vi "WildBugChilGru_V2.0.1.vi"() -> ()   [LabVIEW 2014]
uses:
  <vilib>/Utility/miscctls.llb/LVPointTypeDef.ctl
  <vilib>/Utility/xml.llb/Read From XML File(string).vi
  <vilib>/Utility/xml.llb/Write to XML File(string).vi
  <vilib>/Instr/_visa.llb/VISA Configure Serial Port (Instr).vi
  <vilib>/Analysis/3filter.llb/IIR Filter (DBL).vi
  <vilib>/gmath/NI_Gmath.lvlib
  <vilib>/Analysis/NI_AALBase.lvlib
panel:
  out "Hinterrad (Tacho)\n[km/h]":dbl(knob) scale=0.0..150.0 scale format="%#.0f"
  out "Welle (Tacho)\n[1/min]":cluster{dbl, dbl}(knob) scale=0.0..14000.0
  out "XY-Graph":cluster{dbl[], dbl[]}[](graph)
  in  "Registerkarte":T1(tab)
  in  "Zündung [Imp/U]":dbl=1.0
  in  "Übersetzung ermitteln aus":T2(ring)
  in  "Getriebe [1:]":dbl=4.0
  in  "Reifenumfang [m]":dbl=1.2
  in  "Dauer [s]":dbl=5.0
  in  "nKuWe/nRolle":dbl=1.0 format="%#.3f"
  in  "Lufttemperatur [°C]":dbl
  in  "Luftfeuchtigkeit [%]":dbl=43.8
  in  "Luftdruck [mbar]":dbl=1013.45
  in  "Messung Klimadaten":bool=TRUE
  in  "Gleitender Mittelwert":u8=35
  in  "Differenzenquotient":u8=12
  in  "n vom Gas [1/min]":dbl=5000.0
  in  "Rollengeber [Inkr/U]":u16=200
  in  "Rollenumfang [m]":dbl=0.613
  in  "Rollenträgheit [kgm²]":dbl=0.402
  in  "Recalc":bool
  in  "Leistung":bool=TRUE caption="Messung Klimadaten"
  in  "Ende":bool
  out "Datenspeicher":T3={"Fahrzeugdaten"="", "date/time string"="", "Rolle [Inkr/U]"=200, "Rollenumfang [m]"=0.613, "Rollenträgheit [kgm²]"=0.402, "Zündung [Imp/U]"=1.0, "Getriebe [1:]"=4.0, "Reifenumfang [m] "=1.2, "element"=0.0, "Gl. Mittelwert"=35, "Differenzenquotient"=12, "Polynom"=0, "dT [s]"=0.0, "element"=0.0, "Lufttemperatur [°C]"=0.0, "Luftfeuchtigkeit [%]"=43.8, "Luftdruck [mbar]"=1013.45, [], [], "Best Polynomial Fit"=[], [], "Übersetzung ermitteln aus"=0, "[s]"=5.0, "nmin [1/min]"=0.0, "nmax [1/min]"=0.0, "n vom Gas [1/min]"=5000.0, "dT-Array [s]"=[], [], "Boolesch"=TRUE, "Serielle Schnittstelle"="COM6", "nKuWe/nRolle"=1.0}
  out "COM-Fehlerrate":string="0 / 0,0%"
  in  "Konfiguration:":bool
  in  "Speichern":bool
  in  "Drucken":bool
  out "Pmax":string="0,0 PS"
  out "Ergebnis":string
  in  "Fahrzeugdaten":string
  out "Untersetzung\nermittelt":bool
  out "Untersetzung":dbl format="%#.3f"
  in  "Start":bool
  out "Füllstand Lesepuffer":u64(slide)=1 scale=1.0..100.0
  out "Hinterrad\n[km/h]":dbl(knob) scale=0.0..150.0
  out "Welle\n[1/min]":cluster{dbl, dbl}(knob) scale=0.0..14000.0
  out "Lesepuffer":string="\n"
  in  "Serielle Schnittstelle":refnum<visa-resource-name>="COM6"
  out "Untersetzung-Graph":dbl(graph)=198.99999999999997 caption="Untersetzung"
  # "1. n konstant halten\n2. START\n3. n weiter halten\n4. bei GO: Vollgas\n5. vom Gas gehen"
  # "Zündung\nRolle"
  # "Zündung\nRolle"
  # "Untersetzung aus:"
  # "Eingabe <> Messen"
  # "Tacho <> Leistung"
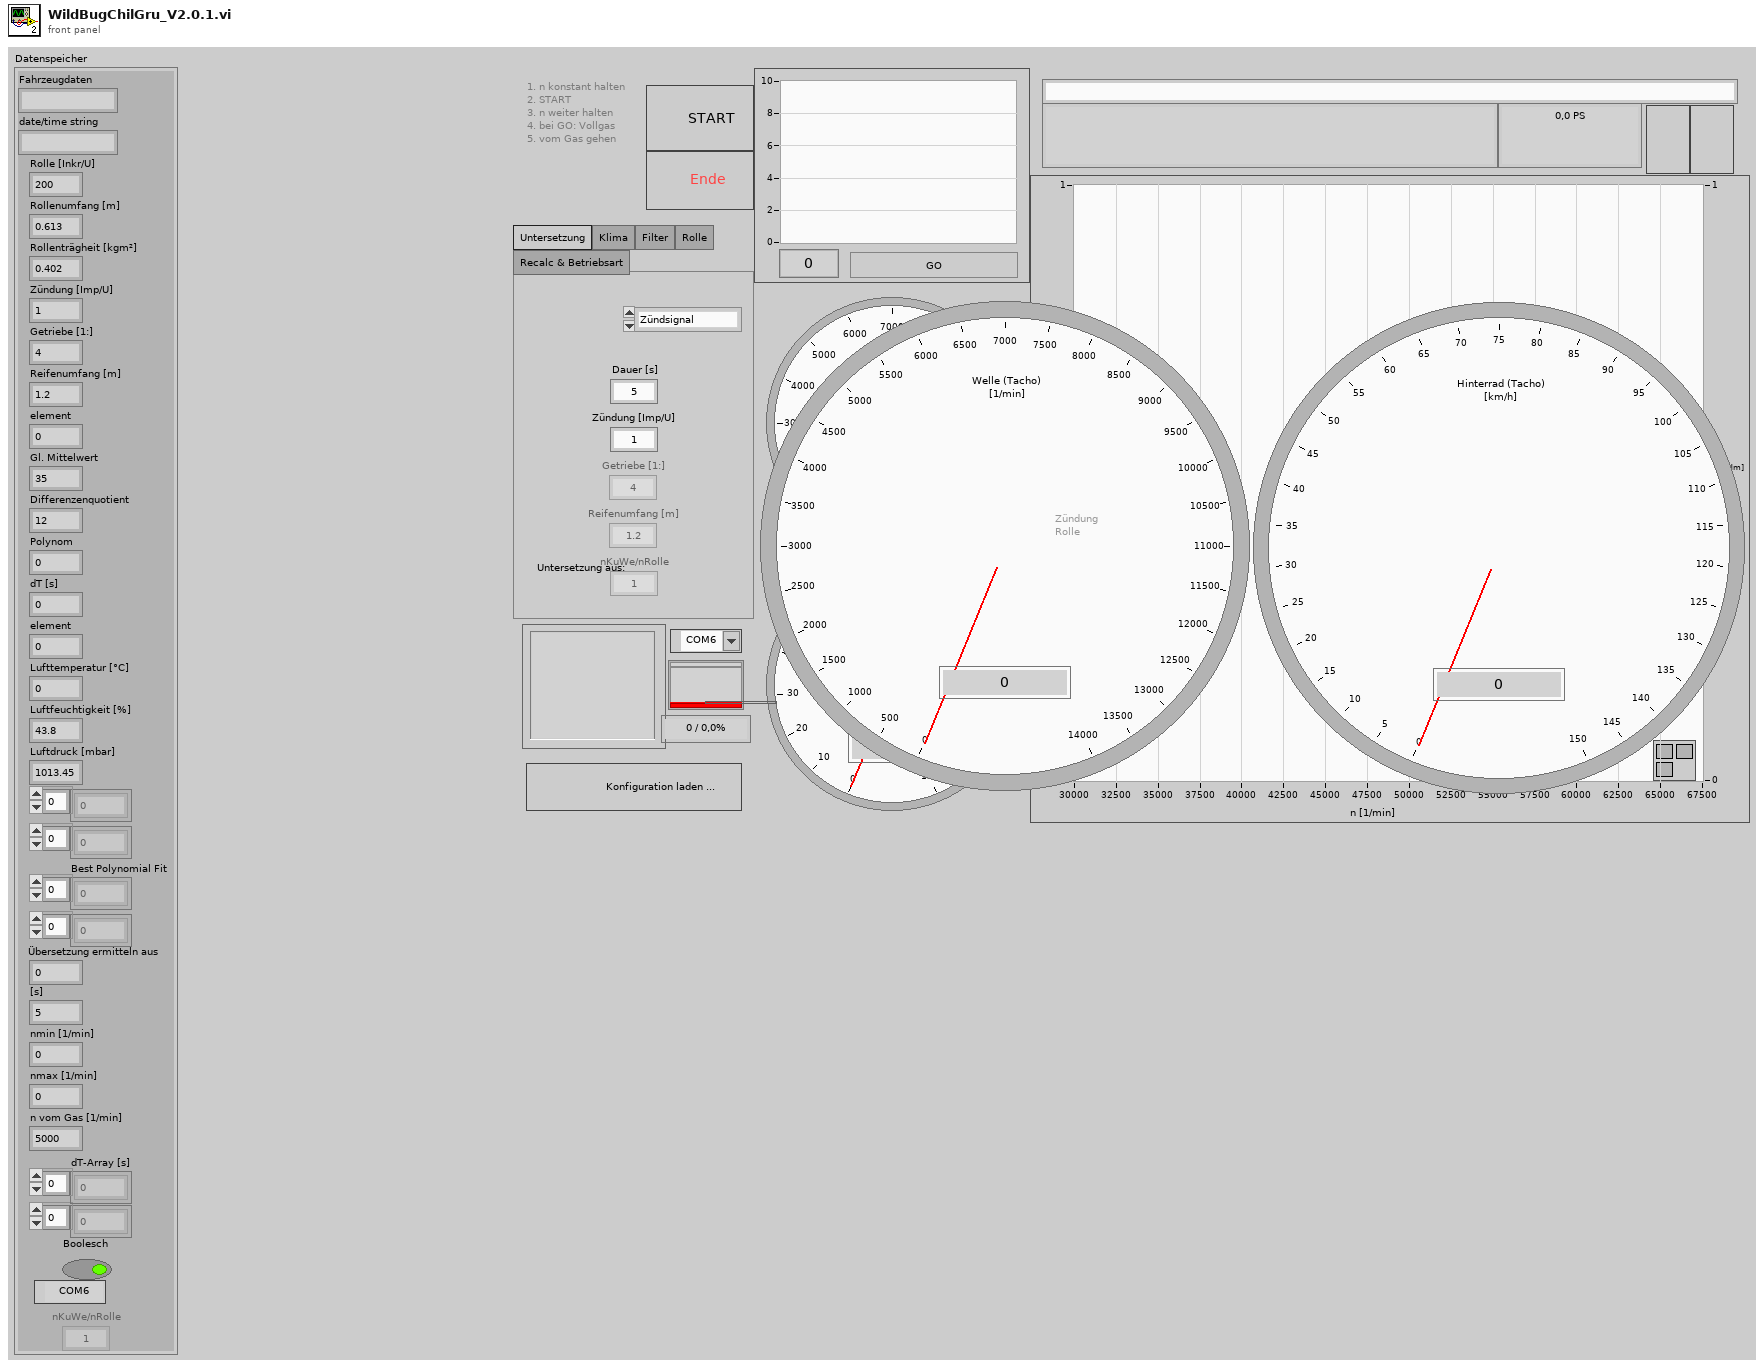
[diagram p1: front panel]
types:
  T1 = enum32{"Untersetzung", "Klima", "Filter", "Rolle", "Recalc & Betriebsart"}
  T2 = enum8{"Zündsignal", "Getriebe & Reifen", "nKuWe / nRolle"}
  T3 = cluster{"Fahrzeugdaten":string, "date/time string":string, "Rolle [Inkr/U]":u16, "Rollenumfang [m]":dbl, "Rollenträgheit [kgm²]":dbl, "Zündung [Imp/U]":dbl, "Getriebe [1:]":dbl, "Reifenumfang [m] ":dbl, "element":dbl, "Gl. Mittelwert":u8, "Differenzenquotient":u8, "Polynom":u8, "dT [s]":dbl, "element":dbl, "Lufttemperatur [°C]":dbl, "Luftfeuchtigkeit [%]":dbl, "Luftdruck [mbar]":dbl, dbl[], dbl[], "Best Polynomial Fit":dbl[], dbl[], "Übersetzung ermitteln aus":u8, "[s]":dbl, "nmin [1/min]":dbl, "nmax [1/min]":dbl, "n vom Gas [1/min]":dbl, "dT-Array [s]":dbl[], i32[], "Boolesch":bool, "Serielle Schnittstelle":refnum<visa-resource-name>, "nKuWe/nRolle":dbl}
  T4 = enum8{"Enabled", "Disabled", "Disabled and Grayed Out"}
  T5 = cluster{"Fahrzeugdaten":string, "date/time string":string, "Rollengeber [Inkr/U]":u16, "Rollenumfang [m]":dbl, "Rollenträgheit [kgm²]":dbl, "Zündung [Imp/U]":dbl, "Getriebe [1:]":dbl, "Reifenumfang [m] ":dbl, "mean value":dbl, "Gleitender Mittelwert":u8, "Differenzenquotient":u8, i32, dbl, "element":dbl, "Lufttemperatur [°C]":dbl, "Luftfeuchtigkeit [%]":dbl, "Luftdruck [mbar]":dbl, dbl[], dbl[], dbl[], dbl[], "Übersetzung ermitteln aus":enum8{"Zündsignal", "Getriebe & Reifen", "nKuWe / nRolle"}, "Dauer [s]":dbl, dbl, dbl, "n vom Gas [1/min]":dbl, dbl[], i32[], "Messung Klimadaten":bool, "VISA resource name out":refnum<visa-resource-name>, "nKuWe/nRolle":dbl}
  T6 = cluster{"Fahrzeugdaten":string, "date/time string":string, "Rolle [Inkr/U]":u16, "Rollenumfang [m]":dbl, "Rollenträgheit [kgm²]":dbl, "Zündung [Imp/U]":dbl, "Getriebe [1:]":dbl, "Reifenumfang [m] ":dbl, "element":dbl, "Gl. Mittelwert":u8, "Differenzenquotient":u8, "Polynom":u8, "element":dbl, "element":dbl, "Lufttemperatur [°C]":dbl, "Luftfeuchtigkeit [%]":dbl, "Luftdruck [mbar]":dbl, dbl[], dbl[], "Best Polynomial Fit":dbl[], dbl[], "Übersetzung ermitteln aus":u8, "[s]":dbl, "nmin [1/min]":dbl, "nmax [1/min]":dbl, "n vom Gas [1/min]":dbl, dbl[], i32[], "Boolesch":bool, "Serielle Schnittstelle":refnum<visa-resource-name>, dbl}
  T7 = typedef "LVPointTypeDef.ctl" = cluster{"Horizontal":i16, "Vertical":i16}
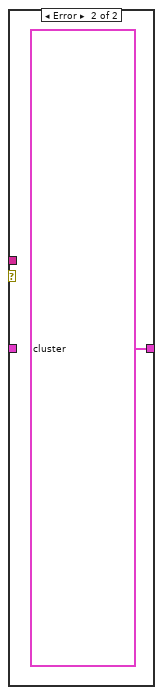
[diagram p2: hidden frame]
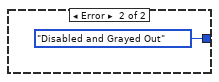
[diagram p3: hidden frame]
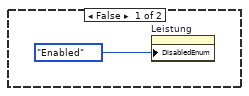
[diagram p4: hidden frame]
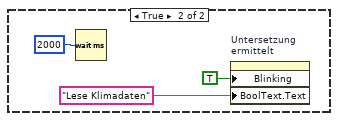
[diagram p5: hidden frame]
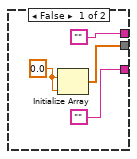
[diagram p8: hidden frame]
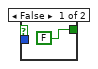
[diagram p9: hidden frame]
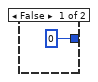
[diagram p11: hidden frame]
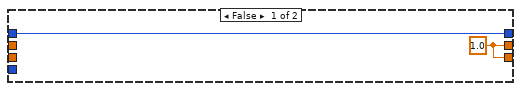
[diagram p13: hidden frame]
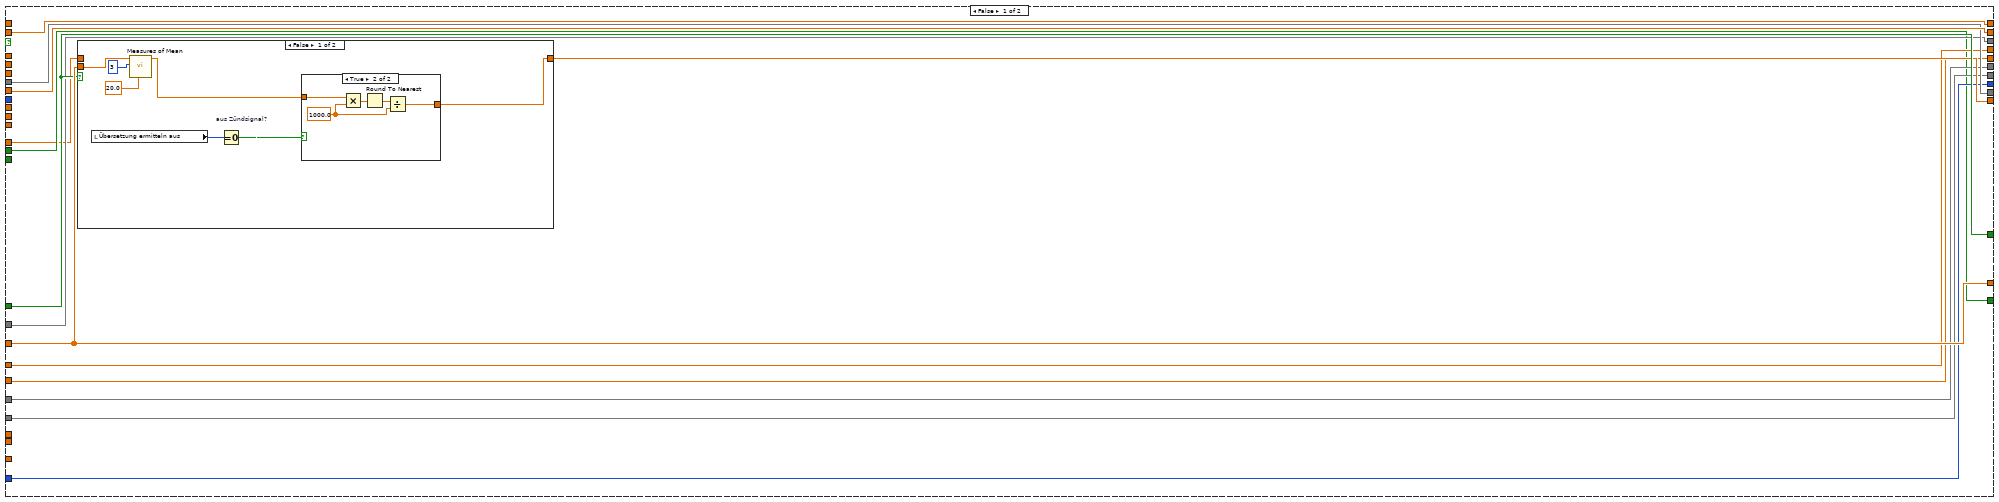
[diagram p14: hidden frame]
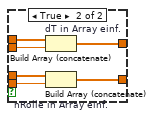
[diagram p17: hidden frame]
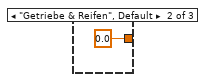
[diagram p20: hidden frame]
diagram:
  n1 = while {
    stop <- w3 stop-if-true
    n2 = Not(x="Leistung") -> (.not. x?=w1:bool)
    n3 = property on="Welle (Tacho)\n[1/min]" class="Drehknopf (strikt)"("Visible"=w1) -> ()  [unwired: 2 in, 2 out]
    n4 = property on="Hinterrad (Tacho)\n[km/h]" class="Drehknopf (strikt)"("Visible"=w1) -> ()  [unwired: 2 in, 2 out]
    n5 = local read "Start"() -> (w4:bool)
    n6 = case shown="True" w4 {
      tunnel: "Leistung" -> [_ w6]
      frame False {
        n7 = property on="Leistung" class="Bool. (strikt)"("DisabledEnum"=T4."Enabled" ("Deaktiviert")) -> ()  [unwired: 2 in, 2 out]
      }
      frame True {
        n8 = flat-sequence {
          tunnel: [w134] -> w120
          tunnel: [w133] -> w119
          tunnel: [w131] -> w118
          tunnel: w6 -> [w129]
          tunnel: w120 -> [w144]
          tunnel: w119 -> [w148]
          tunnel: [0] -> w117
          tunnel: [1.0 ("element")] -> w116
          tunnel: [w146] -> w115
          tunnel: [w158] -> w114
          tunnel: [0] -> w113
          tunnel: [w146] -> w112
          tunnel: [-5] -> w111
          tunnel: [w155] -> w110
          tunnel: [w153] -> w109
          tunnel: [w152] -> w108
          tunnel: [0.0] -> w107
          tunnel: [w144] -> w106
          tunnel: [w148] -> w105
          tunnel: w118 -> [w147]
          tunnel: [w147] -> w104
          tunnel: w117 -> [w184]
          tunnel: [w184] -> w103
          tunnel: w116 -> [w183]
          tunnel: [w183] -> w102
          tunnel: w115 -> [w182]
          tunnel: [w182] -> w101
          tunnel: w114 -> [w181]
          tunnel: [w181] -> w100
          tunnel: w113 -> [w180]
          tunnel: [w180] -> w99
          tunnel: w112 -> [w179]
          tunnel: [w179] -> w98
          tunnel: w111 -> [w178]
          tunnel: [w178] -> w97
          tunnel: w110 -> [w177]
          tunnel: [w177] -> w96
          tunnel: w109 -> [w176]
          tunnel: [w176] -> w95
          tunnel: w108 -> [w175]
          tunnel: [w175] -> w94
          tunnel: w107 -> [w174]
          tunnel: [w174] -> w93
          tunnel: w106 -> [w173]
          tunnel: [w170] -> w92
          tunnel: w105 -> [w172]
          tunnel: [w171] -> w91
          tunnel: w104 -> [w169]
          tunnel: [w169] -> w7
          tunnel: w103 -> [w208]
          tunnel: [w208] -> w90
          tunnel: w102 -> [w207]
          tunnel: [w207] -> w89
          tunnel: w101 -> [w206]
          tunnel: [w206] -> w88
          tunnel: w100 -> [w205]
          tunnel: [w205] -> w87
          tunnel: w99 -> [w204]
          tunnel: [w204] -> w86
          tunnel: w98 -> [w203]
          tunnel: [w203] -> w85
          tunnel: w97 -> [w202]
          tunnel: [w202] -> w84
          tunnel: w96 -> [w201]
          tunnel: [w201] -> w83
          tunnel: w95 -> [w200]
          tunnel: [w200] -> w82
          tunnel: w94 -> [w199]
          tunnel: [w199] -> w81
          tunnel: w93 -> [w198]
          tunnel: [w198] -> w80
          tunnel: w92 -> [w197]
          tunnel: [w197] -> w79
          tunnel: w91 -> [w196]
          tunnel: [w196] -> w78
          tunnel: [w194] -> w8
          tunnel: w7 -> [w194]
          tunnel: w90 -> [w224]
          tunnel: [w224] -> w77
          tunnel: w89 -> [w223]
          tunnel: [w223] -> w76
          tunnel: w88 -> [w222]
          tunnel: [w222] -> w75
          tunnel: w87 -> [w221]
          tunnel: [w221] -> w74
          tunnel: w86 -> [w220]
          tunnel: [w220] -> w73
          tunnel: w85 -> [w219]
          tunnel: [w219] -> w72
          tunnel: w84 -> [w218]
          tunnel: [w218] -> w71
          tunnel: w83 -> [w217]
          tunnel: [w217] -> w70
          tunnel: w82 -> [w216]
          tunnel: [w216] -> w69
          tunnel: w81 -> [w215]
          tunnel: [w215] -> w68
          tunnel: w80 -> [w214]
          tunnel: [w214] -> w67
          tunnel: w79 -> [w213]
          tunnel: [w212] -> w66
          tunnel: w78 -> [w210]
          tunnel: [w211] -> w65
          tunnel: w8 -> [w209]
          tunnel: w77 -> [w303]
          tunnel: w76 -> [w302]
          tunnel: w75 -> [w301]
          tunnel: w74 -> [w300]
          tunnel: w73 -> [w299]
          tunnel: w72 -> [w298]
          tunnel: w71 -> [w297]
          tunnel: w70 -> [w296]
          tunnel: w69 -> [w295]
          tunnel: w68 -> [w294]
          tunnel: w67 -> [w293]
          tunnel: w66 -> [w259]
          tunnel: [w303] -> w64
          tunnel: [w302] -> w63
          tunnel: [w301] -> w62
          tunnel: [w300] -> w61
          tunnel: [w299] -> w60
          tunnel: [w298] -> w59
          tunnel: [w297] -> w58
          tunnel: [w296] -> w57
          tunnel: [w295] -> w56
          tunnel: [w294] -> w55
          tunnel: [w293] -> w54
          tunnel: [w259] -> w53
          tunnel: [w258] -> w52
          tunnel: [w292] -> w51
          tunnel: [w291] -> w50
          tunnel: [w290] -> w49
          tunnel: ["Gleitender Mittelwert"] -> w48
          tunnel: w65 -> [w258]
          tunnel: [w252] -> w11
          tunnel: [w251] -> w10
          tunnel: [w312] -> w20
          tunnel: [w313] -> w21
          tunnel: [w314] -> w22
          tunnel: [w315] -> w23
          tunnel: [w306] -> w18
          tunnel: [w305] -> w19
          tunnel: [w316] -> w24
          tunnel: [w317] -> w25
          tunnel: [w318] -> w27
          tunnel: [w319] -> _
          tunnel: [w320] -> w29
          tunnel: [w321] -> w30
          tunnel: [w322] -> w43
          tunnel: [w323] -> w9
          tunnel: [w324] -> w45
          tunnel: [w325] -> w46
          tunnel: [w326] -> w47
          tunnel: w64 -> [w326]
          tunnel: w63 -> [w325]
          tunnel: w62 -> [w324]
          tunnel: w61 -> [w323]
          tunnel: w60 -> [w322]
          tunnel: w59 -> [w321]
          tunnel: w58 -> [w320]
          tunnel: w57 -> [w319]
          tunnel: w56 -> [w318]
          tunnel: w55 -> [w317]
          tunnel: w54 -> [w316]
          tunnel: w53 -> [w308]
          tunnel: w52 -> [w307]
          tunnel: w51 -> [w315]
          tunnel: w50 -> [w314]
          tunnel: w49 -> [w313]
          tunnel: w48 -> [w312]
          frame #0 {
            w139 = u16 0 items=["None", "XON/XOFF", "RTS/CTS", "XON/XOFF & RTS/CTS", "DTR/DSR", "XON/XOFF & DTR/DSR"] ("flow control (0:none)")
            w140 = u16 10 items=["1.0"=10, "1.5"=15, "2.0"=20] ("stop bits (10: 1 bit)")
            w132 = FALSE  # Enable Termination Char (T)
            w135 = u32 10000  # timeout (10sec)
            n9 = call-poly "VISA Configure Serial Port"("VISA resource name"="Serielle Schnittstelle", "timeout (10sec)"=w135, "Enable Termination\nChar (T)"=w132, "baud rate (9600)"=u32 115200 ("baudrate (250000)"), "data bits (8)"=u16 8, "parity (0:none)"=enum16{"None", "Odd", "Even", "Mark", "Space"}."None", "stop bits (10: 1 bit)"=w140, "flow control (0:none)"=w139) -> ("VISA resource name out"=w137:refnum<visa-resource-name>, "error out"=w136:errorcluster)  [unwired: 6 in]
            n10 = VISA Clear(VISA resource name=w137, error in (no error)=w136) -> (VISA resource name out=w134:refnum<visa-resource-name>, error out=w133:errorcluster)
            n11 = And(x="Messung Klimadaten", y=w129) -> (x .and. y?=w131:bool)
          }
          frame #1 {
            w145 = T4."Disabled and Grayed Out" ("Deaktiviert")
            w151 = 0.0  # Graphen löschen
            w154 = 0
            w159 = 0.0
            w146 = FALSE
            w152 = ""
            n12 = case shown="False" w147 {
              frame False {
                n13 = property on="Untersetzung\nermittelt" class="Bool. (strikt)"("Blinking"=TRUE ("Blinkend"), "BoolText.Text"="Initialisiere" ("Beschriftung.Text")) -> ()  [unwired: 2 in, 2 out]
              }
              frame True {
                n14 = Wait (ms)(milliseconds to wait=u32 2000 ("Zu wartende ms")) -> ()  [unwired: 1 out]
                n15 = property on="Untersetzung\nermittelt" class="Bool. (strikt)"("Blinking"=TRUE ("Blinkend"), "BoolText.Text"="Lese Klimadaten" ("Beschriftung.Text")) -> ()  [unwired: 2 in, 2 out]
              }
            }
            n16 = Build Array(w151) -> (w150:dbl[])
            n17 = property on="Drucken" class="Bool. (strikt)"("DisabledEnum"=w145) -> ()  [unwired: 2 in, 2 out]
            n18 = property on="Übersetzung ermitteln aus" class="Enum (strikt)"("DisabledEnum"=w145) -> ()  [unwired: 2 in, 2 out]
            n19 = property on="Konfiguration:" class="Bool. (strikt)"("DisabledEnum"=w145) -> ()  [unwired: 2 in, 2 out]
            n20 = property on="Ende" class="Bool. (strikt)"("DisabledEnum"=w145) -> ()  [unwired: 2 in, 2 out]
            n21 = property on="Speichern" class="Bool. (strikt)"("DisabledEnum"=w145) -> ()  [unwired: 2 in, 2 out]
            n22 = property on="Untersetzung-Graph" class="SVDiagr (strikt)"("History Data"=w150) -> ()  [unwired: 2 in, 2 out]
            n23 = local write "Pmax"(w152) -> ()
            n24 = local write "COM-Fehlerrate"(w152) -> ()
            n25 = local write "Ergebnis"(w152) -> ()
            n26 = property on="Leistung" class="Bool. (strikt)"("DisabledEnum"=w145) -> ()  [unwired: 2 in, 2 out]
            n27 = Initialize Array(w159, w159) -> (w158:dbl[])
            n28 = Initialize Array(0.0 ("y"), 0) -> (w155:dbl[])
            n29 = Initialize Array(w154, w154) -> (w153:i32[])
          }
          frame #2 {
            n30 = case shown="True" w169 {
              tunnel: w173 -> [w186 w190]
              tunnel: w172 -> [w185 w189]
              tunnel: [w185 w188] -> w171
              tunnel: [w186 w187] -> w170
              frame False {
              }
              frame True {
                n31 = Concatenate Strings("e" ("String"), "\n") -> (w193:string)
                n32 = VISA Write(VISA resource name=w190, write buffer=w193, error in (no error)=w189) -> (VISA resource name out=w187:refnum<visa-resource-name>, error out=w188:errorcluster)  [unwired: 1 out]
              }
            }
          }
          frame #3 {
            n33 = Wait (ms)(milliseconds to wait=u32 500 ("Zu wartende ms")) -> ()  [unwired: 1 out]
          }
          frame #4 {
            n34 = case shown="True" w209 {
              tunnel: w213 -> [w226 w247]
              tunnel: [w226 w246] -> w212
              tunnel: [w225 w245] -> w211
              tunnel: w210 -> [w225 w244]
              frame False {
              }
              frame True {
                w229 = ";" ("Regulärer Ausdruck")
                n35 = property class="Instr"(reference=w247, error in=w244) -> (reference out=w250:refnum<visa-resource-name>, error out=w249:errorcluster, "Serial Settings:Number of Bytes at Serial Port"=w248:u32)
                n36 = VISA Read(VISA resource name=w250, byte count=w248, error in (no error)=w249) -> (VISA resource name out=w246:refnum<visa-resource-name>, read buffer=w241:string, error out=w245:errorcluster)  [unwired: 1 out]
                n37 = Search and Replace String(replace all?=TRUE ("Alle ersetzen? (F)"), input string=w241, search string="." ("Such-String"), replace string="," ("Ersetzungs-String (\"\")")) -> (result string=w234:string)  [unwired: 4 in, 3 out]
                n38 = Match Pattern(string=w234, regular expression=w229) -> (before substring=w232:string, after substring=w233:string)  [unwired: 1 in, 2 out]
                n39 = Match Pattern(string=w233, regular expression=w229) -> (before substring=w231:string, after substring=w230:string)  [unwired: 1 in, 2 out]
                n40 = Fract/Exp String To Number(string=w232, offset=0 ("Offset")) -> (number=w240:dbl)  [unwired: 2 in, 1 out]
                n41 = local write "Lufttemperatur [°C]"(w240) -> ()
                n42 = Fract/Exp String To Number(string=w231) -> (number=w237:dbl)  [unwired: 3 in, 1 out]
                n43 = Match Pattern(string=w230, regular expression=w229) -> (before substring=w228:string)  [unwired: 1 in, 3 out]
                n44 = Fract/Exp String To Number(string=w228) -> (number=w239:dbl)  [unwired: 3 in, 1 out]
                n45 = Divide(x=w237, y=100.0 ("x")) -> (x/y=w238:dbl)
                n46 = local write "Luftdruck [mbar]"(w238) -> ()
                n47 = local write "Luftfeuchtigkeit [%]"(w239) -> ()
              }
            }
          }
          frame #5 {
            n48 = Wait (ms)(milliseconds to wait=u32 2000 ("Zu wartende ms")) -> ()  [unwired: 1 out]
            n49 = Add(x="Lufttemperatur [°C]", y=273.15) -> (x+y=w274:dbl)
            n50 = Divide ("M_Welle [Nm]")(x=300.0, y=w274) -> (x/y=w277:dbl)
            n51 = Multiply(x="Luftfeuchtigkeit [%]", y=0.01) -> (x*y=w287:dbl)
            n52 = Divide ("M_Welle [Nm]")(x=w274, y=293.15) -> (x/y=w272:dbl)
            n53 = Multiply(x=w287, y=240800000000.0) -> (x*y=w262:dbl)
            n54 = Power Of X(1:w277, 2:5.0) -> (0:w275:dbl)
            n55 = Multiply(x=w262, y=w275) -> (x*y=w281:dbl)
            n56 = Multiply(x=w277, y=-22.644) -> (x*y=w282:dbl)
            n57 = Power Of X(1:w272, 2:0.5) -> (0:w269:dbl)
            n58 = Exponential(1:w282) -> (0:w280:dbl)
            n59 = Multiply "Dampfdruck"(x=w281, y=w280) -> ()  [unwired: 1 out]
            n60 = Subtract "Bei DIN70200 ist absoluter Druck zu verwenden,\nohne Damprdruck abzuziehen!"(x="Luftdruck [mbar]", y=0.0) -> (x-y=w278:dbl)
            n61 = local read "Differenzenquotient"() -> (w253:u8)
            n62 = Divide ("M_Welle [Nm]")(x=1013.0, y=w278) -> (x/y=w270:dbl)
            n63 = Multiply "Korrekturfaktor DIN 70020"(x=w270, y=w269) -> (x*y=w292:dbl)
            n64 = Divide(x="Gleitender Mittelwert", y=2) -> (x/y=w266:dbl)
            n65 = call <vilib>:"Smoothing Filter Coefficients.vi"("shape"=0, "half-width"=w253, "type"=0) -> ("forward coefficients"=w251:dbl[], "reverse coefficients"=w252:dbl[])  [unwired: 6 in, 1 out]
            n66 = Round Toward -Infinity(1:w266) -> (0:w265:dbl)
            n67 = call <vilib>:"Smoothing Filter Coefficients.vi"("shape"=1, "half-width"=w265, "type"=0) -> ("forward coefficients"=w290:dbl[], "reverse coefficients"=w291:dbl[])  [unwired: 6 in, 1 out]
          }
          frame #6 {
            n68 = Concatenate Strings("m" ("String"), "\n") -> (w311:string)
            n69 = property on="Untersetzung\nermittelt" class="Bool. (strikt)"("Blinking"=FALSE ("Blinkend")) -> ()  [unwired: 2 in, 2 out]
            n70 = VISA Write(VISA resource name=w308, write buffer=w311, error in (no error)=w307) -> (VISA resource name out=w305:refnum<visa-resource-name>, error out=w306:errorcluster)  [unwired: 1 out]
          }
        }
        n71 = while {
          tunnel: w19 -> [w447]
          tunnel: w18 -> [w446]
          shift-right: [w513] -> _
          shift-left: w25 -> [w462]
          shift-right: [w508] -> _
          shift-left: w24 -> [w512]
          shift-right: [w507] -> _
          shift-left: w24 -> [w511]
          shift-right: [w466] -> _
          shift-left: w24 -> [w510]
          shift-right: [w492] -> _
          shift-left: w47 -> [w509]
          shift-right: [w454] -> w32
          shift-left: w46 -> [_]
          shift-right: [w471] -> w36
          shift-left: w24 -> [w441]
          shift-right: [w436] -> w34
          shift-left: w24 -> [w468]
          shift-right: [w467] -> _
          shift-left: w9 -> [w504]
          shift-right: [w439] -> _
          shift-left: w45 -> [w481]
          shift-right: [w448] -> _
          shift-left: w9 -> [_]
          shift-right: [w453] -> _
          shift-left: w9 -> [_]
          shift-right: [w501] -> w35
          shift-left: w9 -> [w499]
          shift-right: [w500] -> _
          shift-left: w9 -> [w498]
          shift-right: [w487] -> w42
          shift-left: w9 -> [w497]
          shift-right: [w491] -> _
          shift-left: w9 -> [w495]
          shift-right: [w490] -> w12
          shift-left: w9 -> [w496]
          shift-right: [w489] -> w41
          shift-left: w9 -> [w494]
          shift-right: [w488] -> w40
          shift-left: w9 -> [w493]
          tunnel: [w486] -> w44
          shift-right: [w482] -> w39
          shift-left: w43 -> [w484]
          tunnel: [w485] -> w15
          tunnel: ["n vom Gas [1/min]"] -> w38
          tunnel: ["Rollenumfang [m]"] -> w37
          tunnel: ["Rollenumfang [m]"] -> w31
          shift-right: [w478] -> _
          shift-left: w30 -> [w445]
          shift-right: [w472] -> _
          shift-left: w29 -> [w477]
          shift-right: [w473] -> _
          shift-left: w24 -> [w476]
          shift-right: [w474] -> _
          shift-left: w24 -> [w475]
          shift-right: [w444] -> w28
          shift-left: w9 -> [w470]
          shift-right: [w465] -> _
          shift-left: _ -> [w464]
          shift-right: [w469] -> w26
          shift-left: w27 -> [w463]
          tunnel: [w461] -> w16
          tunnel: w23 -> [w454]
          tunnel: w22 -> [w448]
          tunnel: w21 -> [w453]
          tunnel: w20 -> [w452]
          tunnel: w11 -> [w443]
          tunnel: w10 -> [w442]
          stop <- w486 stop-if-true
          n72 = property class="Instr"(reference=w447, error in=w446) -> (reference out=w457:refnum<visa-resource-name>, error out=w456:errorcluster, "Serial Settings:Number of Bytes at Serial Port"=w459:u32)
          n73 = Greater?(x=w459, y=u32 1 ("min. Bytes")) -> (0:w455:bool)
          n74 = case shown="True" w455 {
            tunnel: w459 -> [_ w519]
            tunnel: [u32 0 ("Bytes at Port") w519] -> w458
            frame False {
            }
            frame True {
            }
          }
          n75 = case shown="1.." w458 {
            selector: w458 -> [_ w805]
            tunnel: [w755 w799] -> w485
            tunnel: [w754 w800] -> w461
            tunnel: [w759 w801] -> w507
            tunnel: [w760 w798] -> w508
            tunnel: w462 -> [w761 w796]
            tunnel: [w761 w794] -> w513
            tunnel: w512 -> [w760 w786]
            tunnel: w511 -> [w759 w785]
            tunnel: [w756 w784] -> w466
            tunnel: w510 -> [w756 w783]
            tunnel: w509 -> [w758 _]
            tunnel: [w758 w766] -> w492
            tunnel: [w757 w772] -> w465
            tunnel: w464 -> [w757 w771]
            tunnel: w457 -> [w754 w763]
            tunnel: w456 -> [w755 w762]
            frame 0, Default {
              # "No data in from serial port - Nothing to do."
            }
            frame 1.. {
              # "Hz Drum"
              n76 = VISA Read(VISA resource name=w763, byte count=w805, error in (no error)=w762) -> (VISA resource name out=w800:refnum<visa-resource-name>, read buffer=w797:string, error out=w799:errorcluster)  [unwired: 1 out]
              n77 = Concatenate Strings(w796, w797) -> (w768:string)
              "Lesepuffer" <- w768
              n78 = Spreadsheet String To Array(delimiter (Tab)="\n" ("regular expression"), format string="%s" ("regular expression"), spreadsheet string=w768, array type (2D Dbl)=string[] [] ("Array 2")) -> (array=w777:string[])
              n79 = Match Pattern(string=w768, regular expression="[\\n]") -> (before substring=w775:string, after substring=w795:string, offset past match=w809:i32)  [unwired: 1 in, 1 out]
              n80 = Array Size(array=w777) -> (size(s)=w781:i32)
              n81 = Match Pattern(string=w775, regular expression="[;]") -> (before substring=w773:string, after substring=w774:string, offset past match=w770:i32)  [unwired: 1 in, 1 out]
              n82 = Subtract "aktuelle Zeilenanzahl"(x=w781, y=1) -> (x-y=w766:i32)
              n83 = property on="Füllstand Lesepuffer" class="Schieber (strikt)"() -> ("Scale.Maximum"=w765:dbl)  [unwired: 2 in, 2 out]
              n84 = Match Pattern(string=w774, regular expression="[;]") -> (before substring=w804:string, after substring=w807:string, offset past match=w792:i32)  [unwired: 1 in, 1 out]
              n85 = Match Pattern(string=w807, regular expression="[;]") -> (before substring=w803:string, after substring=w802:string, offset past match=w790:i32)  [unwired: 1 in, 1 out]
              n86 = Greater Or Equal To 0?(x=w770) -> (x >= 0?=w769:bool)
              n87 = Greater?(x=w766, y=w765) -> (0:w767:bool)
              n88 = Greater Or Equal To 0?(x=w790) -> (x >= 0?=w789:bool)
              n89 = Greater Or Equal To 0?(x=w792) -> (x >= 0?=w791:bool)
              n90 = Greater Or Equal To 0?(x=w809) -> (x >= 0?=w793:bool)
              n91 = Select(t=w766, s=w767, f=w765) -> (s? t:f=w764:dbl)
              n92 = Build Array(w793, w791, w769, w789) -> (w788:bool[])
              n93 = property on="Füllstand Lesepuffer" class="Schieber (strikt)"("Scale.Maximum"=w764) -> ()  [unwired: 2 in, 2 out]
              n94 = And Array Elements(Boolean array=w788) -> (logical AND=w787:bool)
              n95 = case shown="True" w787 {
                tunnel: w804 -> [_ w820]
                tunnel: w803 -> [_ w825]
                tunnel: w802 -> [_ w824]
                tunnel: [w813 w823] -> w801
                tunnel: [w814 w822] -> w798
                tunnel: w795 -> [_ w821]
                tunnel: [w815 w821] -> w794
                tunnel: w768 -> [w815 _]
                tunnel: w786 -> [w814 _]
                tunnel: w785 -> [w813 _]
                tunnel: [w812 w819] -> w784
                tunnel: w783 -> [w812 _]
                tunnel: w773 -> [_ w818]
                tunnel: [w811 w816] -> w772
                tunnel: w771 -> [w811 _]
                frame False {
                }
                frame True {
                  # "Cyclecounter"
                  # "Hz ComLevel"
                  # "ComLevel\nLevel 10 =   6Hz \nLevel 5 =   12Hz \nLevel 4 =   15Hz\nLevel 3 =   20Hz\nLevel 2 =   33Hz\nLevel 1 =   62Hz"
                  # "Hz Drum"
                  # "Hz Engine"
                  # "t4m"
                  n96 = Fract/Exp String To Number(string=w818) -> (number=w817:dbl)  [unwired: 3 in, 1 out]
                  n97 = Fract/Exp String To Number(string=w824) -> (number=w823:dbl)  [unwired: 3 in, 1 out]
                  n98 = Fract/Exp String To Number(string=w820) -> (number=w819:dbl)  [unwired: 3 in, 1 out]
                  n99 = To Long Integer(number=w817) -> (32bit integer=w816:i32)
                  n100 = Fract/Exp String To Number(string=w825) -> (number=w822:dbl)  [unwired: 3 in, 1 out]
                }
              }
            }
          }
          "Füllstand Lesepuffer" <- w492
          n101 = Not Equal?(x=w464, y=w465) -> (x != y?=w449:bool)
          n102 = case shown="True" w449 {
            tunnel: w477 -> [w523 w534]
            tunnel: [w523 w546] -> w472
            tunnel: w476 -> [w522 w545]
            tunnel: [w522 w531] -> w473
            tunnel: w475 -> [w521 w544]
            tunnel: [w521 w532] -> w474
            tunnel: w465 -> [_ w530]
            tunnel: w463 -> [w520 w529]
            tunnel: [w520 w533] -> w469
            frame False {
            }
            frame True {
              n103 = Build Array (concatenate)(w529, w530) -> (w533:i32[])
              n104 = Greater Or Equal To 0?(x=w534) -> (x >= 0?=w535:bool)
              n105 = case shown="True" w535 {
                tunnel: [w547 w558] -> w531
                tunnel: [w547 w559] -> w532
                tunnel: [w548 w550] -> w546
                tunnel: w545 -> [_ w552]
                tunnel: w544 -> [_ w560]
                tunnel: w530 -> [w548 w549]
                tunnel: w534 -> [_ w550]
                frame False {
                  w547 = 1.0
                }
                frame True {
                  w556 = 65536.0
                  n106 = Add(x=w550, y=w552) -> (x+y=w551:dbl)
                  n107 = Increment(x=w560) -> (x+1=w559:dbl)
                  n108 = Divide(x=w551, y=w556) -> (x/y=w561:dbl)
                  n109 = Round Toward -Infinity(1:w561) -> (0:w557:dbl)
                  n110 = Multiply(x=w557, y=w556) -> (x*y=w555:dbl)
                  n111 = Add(x=w555, y=w549) -> (x+y=w554:dbl)
                  n112 = Increment(x=w554) -> (x+1=w553:dbl)
                  n113 = Subtract(x=w553, y=w550) -> (x-y=w558:dbl)
                }
              }
              n114 = Subtract(x=w531, y=w532) -> (x-y=w526:dbl)
              n115 = Decrement(x=w526) -> (x-1=w525:dbl)
              n116 = Max & Min(x=0, y=w525) -> (max(x,y)=w524:dbl)  [unwired: 1 out]
              n117 = Divide(x=w524, y=w531) -> (x/y=w538:dbl)
              n118 = Greater Than 0?(x=w524) -> (x > 0?=w528:bool)
              n119 = Select(t=u32 16711680, s=w528, f=u32 0) -> (s? t:f=w539:u32)
              n120 = Multiply(x=w538, y=100.0) -> (x*y=w536:dbl)
              n121 = Format Into String(format string="%d / %.1f%%" ("Format-String"), w524, w536) -> (resulting string=→"COM-Fehlerrate":string)  [unwired: 2 in, 1 out]
              n122 = property on="COM-Fehlerrate" class="Str"("Text.TextColor"=w539) -> ()  [unwired: 2 in, 2 out]
            }
          }
          n123 = case "Case-Struktur" shown="True" w449 {
            tunnel: w508 -> [w735 w747]
            tunnel: w507 -> [w734 w746]
            tunnel: [w735 w745] -> w506
            tunnel: [w734 w744] -> w505
            tunnel: w466 -> [_ w739]
            tunnel: w441 -> [w733 _]
            tunnel: [w733 w738] -> w471
            tunnel: w468 -> [_ w743]
            tunnel: "Rollenumfang [m]" -> [_ w742]
            frame False {
            }
            frame True {
              w753 = 60.0 ("y")
              n124 = Reciprocal "Abtastzeit [s]"(x=w739) -> (1/x=w738:dbl)
              n125 = Divide "R [1/s]"(x=w746, y="Rollengeber [Inkr/U]") -> (x/y=w752:dbl)
              n126 = Divide(x=w747, y="Zündung [Imp/U]") -> (x/y=w750:dbl)
              n127 = Multiply "nZ gemessen [1/min]"(x=w750, y=w753) -> (x*y=w745:dbl)
              n128 = Multiply "nR [1/min]"(x=w753, y=w752) -> (x*y=w744:dbl)
              n129 = Multiply "nZ berechnet [1/min]"(x=w744, y=w743) -> (x*y=w751:dbl)
              n130 = Multiply "[m/min]"(x=w744, y=w742) -> (x*y=w748:dbl)
              n131 = Multiply "[km/h]"(x=w748, y=0.06) -> (x*y=→"Hinterrad\n[km/h]" →"Hinterrad (Tacho)\n[km/h]":dbl)
              n132 = Bundle(w745, w751) -> (→"Welle\n[1/min]" →"Welle (Tacho)\n[1/min]":cluster{dbl, dbl})  [unwired: 1 in]
            }
          }
          n133 = case shown="True" w449 {
            tunnel: w506 -> [_ w654]
            tunnel: w505 -> [_ w653]
            tunnel: "Rollenumfang [m]" -> [_ w657]
            tunnel: [w573 w628] -> w436
            tunnel: w468 -> [w562 w628]
            tunnel: w481 -> [w574 w596]
            tunnel: w504 -> [w575 w660]
            tunnel: [w574 w620] -> w439
            tunnel: [w575 w659] -> w467
            tunnel: w448 -> [_ w656]
            tunnel: w453 -> [_ w655]
            tunnel: [w572 w591] -> w501
            tunnel: [w571 w600] -> w500
            tunnel: w499 -> [w572 w652]
            tunnel: w498 -> [w571 _]
            tunnel: w452 -> [_ w609]
            tunnel: [w570 w634] -> w487
            tunnel: w497 -> [w570 _]
            tunnel: [w569 w599] -> w491
            tunnel: w495 -> [w569 _]
            tunnel: [w568 w635] -> w490
            tunnel: w496 -> [w568 _]
            tunnel: [w567 w646] -> w489
            tunnel: w494 -> [w567 _]
            tunnel: [w566 w645] -> w488
            tunnel: w493 -> [w566 _]
            tunnel: w454 -> [_ w638]
            tunnel: w484 -> [w565 w633]
            tunnel: "n vom Gas [1/min]" -> [_ w622]
            tunnel: [w565 w632] -> w482
            tunnel: w481 -> [_ w631]
            tunnel: w445 -> [w564 w627]
            tunnel: [w564 w626] -> w478
            tunnel: w471 -> [_ w625]
            tunnel: [w563 w592] -> w444
            tunnel: w470 -> [w563 w624]
            tunnel: w443 -> [_ w607]
            tunnel: w442 -> [_ w606]
            frame False {
              n134 = case shown="False" w574 {
                tunnel: w575 -> [w582 _]
                tunnel: [w576 w589] -> w573
                tunnel: w562 -> [_ w589]
                frame False {
                  n135 = local read "Übersetzung ermitteln aus"() -> (w579:T2)
                  n136 = call <vilib>:"Measures of Mean.vi"("percent (trim)"=20.0, "type"=3, "x array"=w582) -> ("mean value"=w577:dbl)  [unwired: 7 in, 1 out]
                  n137 = Equal To 0? "aus Zündsignal?"(x=w579) -> (x = 0?=w578:bool)
                  n138 = case shown="True" w578 {
                    tunnel: w577 -> [w583 w588]
                    tunnel: [w583 w584] -> w576
                    frame False {
                    }
                    frame True {
                      w585 = 1000.0
                      n139 = Multiply(x=w588, y=w585) -> (x*y=w587:dbl)
                      n140 = Round To Nearest(number=w587) -> (nearest integer value=w586:dbl)
                      n141 = Divide(x=w586, y=w585) -> (x/y=w584:dbl)
                    }
                  }
                }
                frame True {
                }
              }
            }
            frame True {
              w641 = 0.00135962  # [W] in [PS]
              w648 = 0.10471975511965978  # 2*Pi/60
              n142 = local read "Leistung"() -> (w594:bool)
              n143 = Not(x=w596) -> (.not. x?=w595:bool)
              n144 = local read "Differenzenquotient"() -> (w605:u8)
              n145 = Or(x=w594, y=w595) -> (x .or. y?=w593:bool)
              n146 = case shown="False" w593 {
                tunnel: w653 -> [_ w668]
                tunnel: w652 -> [w661 w667]
                tunnel: w625 -> [_ w666]
                tunnel: w624 -> [w662 w665]
                tunnel: [w661 w664] -> w591
                tunnel: [w662 w663] -> w592
                frame False {
                }
                frame True {
                  n147 = Build Array (concatenate) "dT in Array einf."(w665, w666) -> (w663:dbl[])
                  n148 = Build Array (concatenate) "nRolle in Array einf."(w667, w668) -> (w664:dbl[])
                }
              }
              n149 = local read "Übersetzung ermitteln aus"() -> (w597:T2)
              n150 = Multiply(x=2, y=w605) -> (x*y=w603:i32)
              n151 = Increment(x=w603) -> (x+1=w601:i32)
              n152 = Index Array(array=w592, index=1 ("Index")) -> (element=w612:dbl)
              n153 = Index Array(array=w591, index=1 ("Index")) -> (element=w618:dbl)
              n154 = case shown="\"Zündsignal\"" w597 {
                tunnel: w654 -> [_ _ w732]
                tunnel: w653 -> [_ _ w731]
                tunnel: [w727 "nKuWe/nRolle" w730] -> w658
                tunnel: w657 -> [w728 _ _]
                frame "Getriebe & Reifen" {
                  n155 = Divide(x=w728, y="Reifenumfang [m]") -> (x/y=w726:dbl)
                  n156 = Multiply(x=w726, y="Getriebe [1:]") -> (x*y=w727:dbl)
                }
                frame "nKuWe / nRolle" {
                }
                frame "Zündsignal" {
                  n157 = Divide(x=w732, y=w731) -> (x/y=w730:dbl)
                }
              }
              n158 = Initialize Array(w612, w601) -> (w610:dbl[])
              n159 = Initialize Array(w618, w609) -> (w617:dbl[])
              n160 = Insert Into Array(array=w591, index=0 ("Index"), new element=w617) -> (w615:dbl[])
              n161 = Insert Into Array(array=w592, index=0 ("Index"), new element=w610) -> (w608:dbl[])
              n162 = call-poly <vilib>:"IIR Filter.vi"("Forward Coefficients"=w655, "Reverse Coefficients"=w656, "X"=w615) -> ("Filtered X"=w614:dbl[])  [unwired: 1 in, 1 out]
              n163 = call-poly <vilib>:"IIR Filter.vi"("Forward Coefficients"=w606, "Reverse Coefficients"=w607, "X"=w608) -> ("Filtered X"=w602:dbl[])  [unwired: 1 in, 1 out]
              n164 = Array Subset "Rolle gefiltert [1/min]"(array=w614, index=w609) -> (w600:dbl[])  [unwired: 1 in]
              n165 = Array Subset "dT gefiltert [s]"(array=w602, index=w601) -> (w598:dbl[])  [unwired: 1 in]
              n166 = case shown="False" w596 {
                selector: w596 -> [_ w723]
                tunnel: w658 -> [w711 _]
                tunnel: w660 -> [w713 w722]
                tunnel: [w708 w723] -> w651
                tunnel: [w712 w722] -> w659
                tunnel: w627 -> [w710 w721]
                tunnel: [w708 w721] -> w626
                tunnel: w597 -> [w707 _]
                frame False {
                  n167 = Build Array (concatenate)(w713, w711) -> (w712:dbl[])
                  n168 = case shown="\"Zündsignal\"" w707 {
                    tunnel: ["Dauer [s]" 0.0 ("Dauer [s]") 0.0] -> w709
                    frame "Zündsignal" {
                      n169 = property on="Untersetzung\nermittelt" class="Bool. (strikt)"("Blinking"=TRUE ("Blinkend"), "BoolText.Text"="Ermittle Übersetzung" ("Boolescher Text.Text")) -> ()  [unwired: 2 in, 2 out]
                    }
                    frame "Getriebe & Reifen", Default {
                    }
                    frame "nKuWe / nRolle" {
                    }
                  }
                  n170 = call "Verstrichene Zeit"("Time Target (s)"=w709, "Reset"=w710) -> ("Time has Elapsed"=w708:bool)  [unwired: 10 in, 7 out]
                  n171 = case shown="True" w708 {
                    frame False {
                    }
                    frame True {
                      n172 = property on="Untersetzung\nermittelt" class="Bool. (strikt)"("Blinking"=FALSE ("Blinkend"), "BoolText.Text"="Go" ("Boolescher Text.Text")) -> ()  [unwired: 2 in, 2 out]
                    }
                  }
                  "Untersetzung-Graph" <- w711
                }
                frame True {
                }
              }
              n173 = Array Size "Array-Größe"(array=w600) -> (size(s)=w649:i32)
              n174 = Square(x=w628) -> (x^2=w647:dbl)
              n175 = Multiply(x=w600, y=w628) -> (x*y=w634:dbl[])
              n176 = Multiply(x=w634, y=w648) -> (x*y=w599:dbl[])
              n177 = Greater?(x=w649, y=w609) -> (0:w650:bool)
              n178 = Divide(x="Rollenträgheit [kgm²]", y=w647) -> (x/y=w639:dbl)
              n179 = Multiply(x=w639, y=w638) -> (x*y=w637:dbl)
              n180 = And(x=w651, y=w650) -> (x .and. y?=w620:bool)
              n181 = Array Size "Array-Größe"(array=w599) -> (size(s)=w590:i32)
              n182 = Initialize Array(0.0 ("y"), 0) -> (w642:dbl[])
              n183 = Decrement(x=w590) -> (x-1=w636:i32)
              n184 = Select(t=w622, s=w620, f=1000000.0) -> (s? t:f=w623:dbl)
              n185 = for {
                N: w590 -> [_]
                tunnel: "Differenzenquotient" -> [w683]
                tunnel: w599 -> [w691]
                tunnel: w636 -> [w682]
                shift-right: [w688] -> w635
                shift-left: w642 -> [w689]
                tunnel: w634 -> [w686] mode=indexing
                tunnel: w633 -> [w675]
                tunnel: w623 -> [w685]
                tunnel: [w676] -> w632
                tunnel: w631 -> [w674]
                tunnel: w598 -> [w671] mode=indexing
                i -> [w672]
                stop <- w669 stop-if-true
                n186 = Subtract(x=w682, y=w683) -> (x-y=w684:i32)
                n187 = Add(x=w672, y=w683) -> (x+y=w698:i32)
                n188 = Subtract(x=w672, y=w683) -> (x-y=w704:i32)
                n189 = Greater Or Equal?(x=w672, y=w683) -> (x >= y?=w679:bool)
                n190 = Greater?(x=w686, y=w685) -> (0:w687:bool)
                n191 = Max & Min(x=w682, y=w698) -> (min(x,y)=w699:i32)  [unwired: 1 out]
                n192 = Max & Min(x=w704, y=0) -> (max(x,y)=w702:i32)  [unwired: 1 out]
                n193 = Subtract(x=w699, y=w672) -> (x-y=w700:i32)
                n194 = Subtract(x=w672, y=w702) -> (x-y=w701:i32)
                n195 = Less Or Equal?(x=w672, y=w684) -> (x <= y?=w680:bool)
                n196 = Max & Min(x=w701, y=w700) -> (min(x,y)=w692:i32)  [unwired: 1 out]
                n197 = Multiply(x=w671, y=2.0) -> (x*y=w673:dbl)
                n198 = Add(x=w672, y=w692) -> (x+y=w697:i32)
                n199 = Subtract(x=w672, y=w692) -> (x-y=w696:i32)
                n200 = Multiply(x=w692, y=w673) -> (x*y=w690:dbl)
                n201 = Index Array(array=w691, index=w697) -> (element=w694:dbl)
                n202 = Index Array(array=w691, index=w696) -> (element=w695:dbl)
                n203 = Subtract(x=w694, y=w695) -> (x-y=w693:dbl)
                n204 = Divide(x=w693, y=w690) -> (x/y=w681:dbl)
                n205 = Less Than 0?(x=w681) -> (x < 0?=w678:bool)
                n206 = Less Or Equal To 0?(x=w675) -> (x <= 0?=w677:bool)
                n207 = Build Array (concatenate)(w689, w681) -> (w688:dbl[])
                n208 = Compound Arithmetic op=AND(w678, w687, w677, w679, w680, w674) -> (w669:bool)
                n209 = case shown="False" w669 {
                  tunnel: w672 -> [_ w706]
                  tunnel: [w705 w706] -> w676
                  tunnel: w675 -> [w705 _]
                  frame False {
                  }
                  frame True {
                  }
                }
              }
              n210 = Multiply(x=w635, y=w637) -> (x*y=w646:dbl[])
              n211 = Multiply(x=w599, y=w646) -> (x*y=w640:dbl[])
              n212 = Multiply(x=w641, y=w640) -> (x*y=w645:dbl[])
            }
          }
          "Untersetzung\nermittelt" <- w439
          n213 = local read "Leistung"() -> (w435:bool)
          n214 = local read "Übersetzung ermitteln aus"() -> (w440:T2)
          n215 = case shown="True" w435 {
            tunnel: [FALSE w516] -> w483
            tunnel: w482 -> [_ w515]
            frame False {
            }
            frame True {
              n216 = Greater Than 0?(x=w515) -> (x > 0?=w516:bool)
            }
          }
          n217 = Select(t=w436, s=w439, f=0.0) -> (s? t:f=→"Untersetzung":dbl)
          n218 = Equal To 0? "aus Zündsignal?"(x=w440) -> (x = 0?=w438:bool)
          n219 = local read "Start"() -> (w451:bool)
          n220 = And(x=w439, y=w438) -> (x .and. y?=w437:bool)
          n221 = case shown="True" w437 {
            tunnel: w436 -> [_ w517]
            frame False {
            }
            frame True {
              n222 = local write "nKuWe/nRolle"(w517) -> ()
            }
          }
          n223 = Not(x=w451) -> (.not. x?=w450:bool)
          n224 = Or(x=w483, y=w450) -> (x .or. y?=w486:bool)
        }
        n225 = VISA Clear(VISA resource name=w16, error in (no error)=w15) -> (VISA resource name out=w13:refnum<visa-resource-name>, error out=w17:errorcluster)
        n226 = VISA Close(VISA resource name=w13, error in (no error)=w17) -> ()  [unwired: 1 out]
        n227 = case shown="True" w44 {
          tunnel: w42 -> [_ w413]
          tunnel: w41 -> [_ w418]
          tunnel: w40 -> [_ w417]
          tunnel: w39 -> [_ w389]
          tunnel: w12 -> [_ w414]
          tunnel: w38 -> [_ w412]
          tunnel: w37 -> [_ w406]
          tunnel: w32 -> [_ w392]
          tunnel: ["" w391] -> w33
          tunnel: w34 -> [_ w390]
          tunnel: ["" w388] -> _
          tunnel: [w368 w376] -> _
          frame False {
            w369 = 0.0
            n228 = Initialize Array(w369, w369) -> (w368:dbl[])
          }
          frame True {
            w387 = 0
            n229 = Array Subset "P"(array=w417, length=w389) -> (w409:dbl[])  [unwired: 1 in]
            n230 = Array Subset "M"(array=w418, length=w389) -> (w410:dbl[])  [unwired: 1 in]
            n231 = Array Subset "alpha"(array=w414, length=w389) -> (w415:dbl[])  [unwired: 1 in]
            n232 = Array Subset "n"(array=w413, length=w389) -> (w411:dbl[])  [unwired: 1 in]
            n233 = property on="Pmax" class="Str"("Text.FontSize"=48) -> ()  [unwired: 2 in, 2 out]
            n234 = property on="Ergebnis" class="Str"("Text.FontSize"=18) -> ()  [unwired: 2 in, 2 out]
            n235 = Array Size(array=w415) -> (size(s)=w416:i32)
            n236 = for {
              N: w416 -> [w434]
              tunnel: w414 -> [w431]
              tunnel: w413 -> [w428]
              tunnel: w412 -> [w425]
              tunnel: [w423] -> w386
              i -> [w429]
              stop <- w424 stop-if-true
              n237 = Decrement(x=w434) -> (x-1=w433:i32)
              n238 = Subtract(x=w433, y=w429) -> (x-y=w423:i32)
              n239 = Index Array(array=w431, index=w423) -> (element=w432:dbl)
              n240 = Index Array(array=w428, index=w423) -> (element=w427:dbl)
              n241 = Less?(x=w427, y=w425) -> (x < y?=w426:bool)
              n242 = Less Or Equal To 0?(x=w432) -> (x <= 0?=w430:bool)
              n243 = And(x=w430, y=w426) -> (x .and. y?=w424:bool)
            }
            n244 = Increment(x=w386) -> (x+1=w385:i32)
            n245 = Array Subset "P"(array=w409, index=w385) -> (w377:dbl[])  [unwired: 1 in]
            n246 = Array Subset "M"(array=w410, index=w385) -> (w376:dbl[])  [unwired: 1 in]
            n247 = Array Subset "n"(array=w411, index=w385) -> (w382:dbl[])  [unwired: 1 in]
            n248 = Bundle(w382, w377) -> (w381:cluster{dbl[], dbl[]})  [unwired: 1 in]
            n249 = Bundle(w382, w376) -> (w380:cluster{dbl[], dbl[]})  [unwired: 1 in]
            n250 = Array Max & Min "nmax [1/min]"(array=w382) -> (max value=w408:dbl)  [unwired: 3 out]
            n251 = Divide(x=w408, y=w390) -> (x/y=w407:dbl)
            n252 = Compound Arithmetic op=MULTIPLY "vmax"(w407, w406, 0.06) -> (w398:dbl)
            n253 = Array Max & Min "Mmax"(array=w376) -> (max value=w383:dbl, max index (indices)=w379:i32)  [unwired: 2 out]
            n254 = Multiply(x=w383, y=1.8) -> (x*y=w374:dbl)
            n255 = Index Array "n(Mmax)"(array=w382, index=w379) -> (element=w399:dbl)
            n256 = Array Max & Min "Pmax"(array=w377) -> (max value=w384:dbl, max index (indices)=w378:i32)  [unwired: 2 out]
            n257 = Round To Nearest(number=w374) -> (nearest integer value=w375:dbl)
            n258 = Multiply(x=w384, y=1.2) -> (x*y=w373:dbl)
            n259 = Build Array(w381, w380) -> (→"XY-Graph":cluster{dbl[], dbl[]}[])
            n260 = local read "Luftfeuchtigkeit [%]"() -> (w402:dbl)
            n261 = local read "Lufttemperatur [°C]"() -> (w401:dbl)
            n262 = local read "Luftdruck [mbar]"() -> (w403:dbl)
            n263 = Round To Nearest(number=w373) -> (nearest integer value=w372:dbl)
            n264 = property on="XY-Graph" class="XYGraph (strikt)"("ActYScl"=1, "YScale.Maximum"=w375, "YScale.Minimum"=w387) -> ()  [unwired: 2 in, 2 out]
            n265 = property on="XY-Graph" class="XYGraph (strikt)"("ActYScl"=w387, "YScale.Maximum"=w372, "YScale.Minimum"=w387) -> ()  [unwired: 2 in, 2 out]
            n266 = Index Array "n(Pmax)"(array=w382, index=w378) -> (element=w404:dbl)
            n267 = Format Into String(format string="%.1f PS" ("Format-String"), w384) -> (resulting string=→"Pmax":string)  [unwired: 2 in, 1 out]
            n268 = Format Date/Time String(time format string (%c)="%x %H:%M ") -> (date/time string=w391:string)  [unwired: 2 in]
            n269 = Format Into String(format string="%.1f PS bei %d 1/min   |   %.1f Nm bei %d 1/min   |   vmax: %d km/h\\nDIN 70020 k =%.3f (%d \\B0C, %d %%, %d mbar)\\n%s" ("Format-String"), w384, w404, w383, w399, w398, w392, w401, w402, w403, w391) -> (resulting string=w388:string)  [unwired: 2 in, 1 out]
            "Ergebnis" <- w388
          }
        }
        n270 = flat-sequence {
          tunnel: w26 -> [w331]
          tunnel: w28 -> [w332]
          tunnel: w31 -> [w333]
          tunnel: w32 -> [w334]
          tunnel: w33 -> [w335]
          tunnel: w34 -> [w336]
          tunnel: w35 -> [w337]
          tunnel: w36 -> [w338]
          tunnel: [w338] -> w128
          tunnel: [w337] -> w127
          tunnel: [w336] -> w126
          tunnel: [w335] -> w125
          tunnel: [w334] -> w124
          tunnel: [w333] -> w123
          tunnel: [w332] -> w122
          tunnel: [w331] -> w121
          tunnel: [w327] -> w14
          tunnel: w13 -> [w327]
          tunnel: w128 -> [w367]
          tunnel: w127 -> [w366]
          tunnel: w126 -> [w365]
          tunnel: w125 -> [w364]
          tunnel: w124 -> [w363]
          tunnel: w123 -> [w362]
          tunnel: w122 -> [w361]
          tunnel: w121 -> [w360]
          tunnel: w14 -> [w342]
          frame #0 {
            w329 = FALSE ("Start [F1]")
            w330 = 0  # Aktivieren
            n271 = local write "Start"(w329) -> ()
            n272 = property on="Speichern" class="Bool. (strikt)"("DisabledEnum"=w330) -> ()  [unwired: 2 in, 2 out]
            n273 = property on="Übersetzung ermitteln aus" class="Enum (strikt)"("DisabledEnum"=w330) -> ()  [unwired: 2 in, 2 out]
            n274 = property on="Konfiguration:" class="Bool. (strikt)"("DisabledEnum"=w330) -> ()  [unwired: 2 in, 2 out]
            n275 = property on="Ende" class="Bool. (strikt)"("DisabledEnum"=w330) -> ()  [unwired: 2 in, 2 out]
            n276 = property on="Drucken" class="Bool. (strikt)"("DisabledEnum"=w330) -> ()  [unwired: 2 in, 2 out]
            n277 = property on="Untersetzung\nermittelt" class="Bool. (strikt)"("BoolText.Text"="GO" ("Boolescher Text.Text"), "Blinking"=w329) -> ()  [unwired: 2 in, 2 out]
            n278 = local write "Untersetzung\nermittelt"(w329) -> ()
          }
          frame #1 {
            w339 = dbl[] []
            w345 = 0.0
            n279 = local read "Übersetzung ermitteln aus"() -> (w348:T2)
            n280 = local read "Rollenträgheit [kgm²]"() -> (w357:dbl)
            n281 = local read "Gleitender Mittelwert"() -> (w353:u8)
            n282 = local read "Messung Klimadaten"() -> (w344:bool)
            n283 = local read "Rollengeber [Inkr/U]"() -> (w358:u16)
            n284 = local read "Differenzenquotient"() -> (w352:u8)
            n285 = local read "Lufttemperatur [°C]"() -> (w351:dbl)
            n286 = local read "Luftfeuchtigkeit [%]"() -> (w350:dbl)
            n287 = local read "Reifenumfang [m]"() -> (w354:dbl)
            n288 = local read "n vom Gas [1/min]"() -> (w346:dbl)
            n289 = local read "Zündung [Imp/U]"() -> (w356:dbl)
            n290 = local read "Luftdruck [mbar]"() -> (w349:dbl)
            n291 = local read "nKuWe/nRolle"() -> (w341:dbl)
            n292 = local read "Getriebe [1:]"() -> (w355:dbl)
            n293 = local read "Dauer [s]"() -> (w347:dbl)
            n294 = Bundle("Fahrzeugdaten"="Fahrzeugdaten", "date/time string"=w364, "Rollengeber [Inkr/U]"=w358, "Rollenumfang [m]"=w362, "Rollenträgheit [kgm²]"=w357, "Zündung [Imp/U]"=w356, "Getriebe [1:]"=w355, "Reifenumfang [m]"=w354, "mean value"=w365, "Gleitender Mittelwert"=w353, "Differenzenquotient"=w352, 0, w367, "element"=w363, "Lufttemperatur [°C]"=w351, "Luftfeuchtigkeit [%]"=w350, "Luftdruck [mbar]"=w349, w366, w339, w339, w339, "Übersetzung ermitteln aus"=w348, "Dauer [s]"=w347, w345, w345, "n vom Gas [1/min]"=w346, w361, w360, "Messung Klimadaten"=w344, "VISA resource name out"=w342, "nKuWe/nRolle"=w341) -> (→"Datenspeicher":T5)  [unwired: 1 in]
          }
        }
      }
    }
    n295 = local read "Ende"() -> (w3:bool)
  }
  n296 = flat-sequence {
    frame #0 {
      n297 = call <vilib>:"Application Directory.vi"() -> ("Application Directory"=w849:path)
      n298 = Build Path(base path=w849, name or relative path="Konfig.xml") -> (appended path=w847:path)
      n299 = call-poly <vilib>:"Read From XML File.vi"("XML File Path"=w847) -> ("error out"=w829:errorcluster, "XML Elements"=w851:string)  [unwired: 8 in, 1 out]
      n300 = property on="Datenspeicher" class="Cluster (strikt)"() -> ("Value"=w850:T3)  [unwired: 2 in, 2 out]
      n301 = case shown="Kein Fehler" w829 {
        tunnel: w851 -> [w854 _]
        tunnel: w850 -> [w853 _]
        tunnel: [w852 T6 {"Fahrzeugdaten"="", "date/time string"="05.02.2017 22:14 ", "Rolle [Inkr/U]"=10, "Rollenumfang [m]"=0.613, "Rollenträgheit [kgm²]"=0.402, "Zündung [Imp/U]"=5.0, "Getriebe [1:]"=5.343, "Reifenumfang [m] "=1.222, "element"=2.0, "Gl. Mittelwert"=35, "Differenzenquotient"=12, "Polynom"=15, "element"=0.01639344262295082, "element"=1.0177230216140456, "Lufttemperatur [°C]"=23.3, "Luftfeuchtigkeit [%]"=43.8, "Luftdruck [mbar]"=1013.45, array[1238 elements], array[1224 elements], "Best Polynomial Fit"=array[1224 elements], array[1224 elements], "Übersetzung ermitteln aus"=0, "[s]"=5.0, "nmin [1/min]"=0.0, "nmax [1/min]"=0.0, "n vom Gas [1/min]"=5000.0, array[1238 elements], array[1238 elements], "Boolesch"=TRUE, "Serielle Schnittstelle"="", 10.0} ("Datenspeicher")] -> w830
        frame No Error {
          n302 = Unflatten From XML(xml string=w854, type=w853) -> (value=w852:T3)  [unwired: 1 in, 1 out]
        }
        frame Error {
        }
      }
      n303 = property on="Datenspeicher" class="Cluster (strikt)"("Value"=w830) -> ()  [unwired: 2 in, 2 out]
      n304 = Unbundle(w830) -> ("Fahrzeugdaten"=w846:string, "Rolle [Inkr/U]"=w845:u16, "Rollenumfang [m]"=w844:dbl, "Rollenträgheit [kgm²]"=w843:dbl, "Zündung [Imp/U]"=w842:dbl, "Getriebe [1:]"=w841:dbl, "Reifenumfang [m]"=w840:dbl, "element"=w828:dbl, "Gl. Mittelwert"=w839:u8, "Differenzenquotient"=w838:u8, "Lufttemperatur [°C]"=w837:dbl, "Luftfeuchtigkeit [%]"=w836:dbl, "Luftdruck [mbar]"=w835:dbl, "Übersetzung ermitteln aus"=w832:u8, "[s]"=w834:dbl, "n vom Gas [1/min]"=w833:dbl, "Boolesch"=w831:bool, "Serielle Schnittstelle"=w827:refnum<visa-resource-name>, "nKuWe/nRolle"=w826:dbl)  [unwired: 12 out]
      n305 = property on="Dauer [s]" class="DigWert (strikt)"("Value"=w834) -> ()  [unwired: 2 in, 2 out]
      n306 = property on="Fahrzeugdaten" class="Str"("Value"=w846) -> ()  [unwired: 2 in, 2 out]
      n307 = property on="Rollengeber [Inkr/U]" class="DigWert (strikt)"("Value"=w845) -> ()  [unwired: 2 in, 2 out]
      n308 = property on="Rollenumfang [m]" class="DigWert (strikt)"("Value"=w844) -> ()  [unwired: 2 in, 2 out]
      n309 = property on="Rollenträgheit [kgm²]" class="DigWert (strikt)"("Value"=w843) -> ()  [unwired: 2 in, 2 out]
      n310 = property on="Zündung [Imp/U]" class="DigWert (strikt)"("Value"=w842) -> ()  [unwired: 2 in, 2 out]
      n311 = property on="Getriebe [1:]" class="DigWert (strikt)"("Value"=w841) -> ()  [unwired: 2 in, 2 out]
      n312 = property on="Reifenumfang [m]" class="DigWert (strikt)"("Value"=w840) -> ()  [unwired: 2 in, 2 out]
      n313 = property on="nKuWe/nRolle" class="DigWert (strikt)"("Value"=w828) -> ()  [unwired: 2 in, 2 out]
      n314 = property on="Gleitender Mittelwert" class="DigWert (strikt)"("Value"=w839) -> ()  [unwired: 2 in, 2 out]
      n315 = property on="Differenzenquotient" class="DigWert (strikt)"("Value"=w838) -> ()  [unwired: 2 in, 2 out]
      n316 = property on="Lufttemperatur [°C]" class="DigWert (strikt)"("Value"=w837) -> ()  [unwired: 2 in, 2 out]
      n317 = property on="Luftfeuchtigkeit [%]" class="DigWert (strikt)"("Value"=w836) -> ()  [unwired: 2 in, 2 out]
      n318 = property on="Luftdruck [mbar]" class="DigWert (strikt)"("Value"=w835) -> ()  [unwired: 2 in, 2 out]
      n319 = property on="Übersetzung ermitteln aus" class="Enum (strikt)"("Val(Sgnl)"=w832) -> ()  [unwired: 2 in, 2 out]
      n320 = property on="n vom Gas [1/min]" class="DigWert (strikt)"("Value"=w833) -> ()  [unwired: 2 in, 2 out]
      n321 = property on="Messung Klimadaten" class="Bool. (strikt)"("Val(Sgnl)"=w831) -> ()  [unwired: 2 in, 2 out]
      n322 = local write "Serielle Schnittstelle"(w827) -> ()
      n323 = property on="nKuWe/nRolle" class="DigWert (strikt)"("Value"=w826) -> ()  [unwired: 2 in, 2 out]
    }
    frame #1 {
      w862 = 2  # Deaktivieren
      w864 = 0.0  # Graphen löschen
      n324 = local read "Serielle Schnittstelle"() -> (w860:refnum<visa-resource-name>)
      n325 = property on="Frontpanel-Position" class="Bereich"("Origin"=T7 {"Horizontal"=8, "Vertical"=6}) -> ()  [unwired: 2 in, 2 out]
      n326 = property on="Füllstand Lesepuffer" class="Schieber (strikt)"("Scale.Maximum"=100) -> ()  [unwired: 2 in, 2 out]
      n327 = property on="Drucken" class="Bool. (strikt)"("DisabledEnum"=w862) -> ()  [unwired: 2 in, 2 out]
      n328 = property on="Speichern" class="Bool. (strikt)"("DisabledEnum"=w862) -> ()  [unwired: 2 in, 2 out]
      n329 = Build Array(w864) -> (w863:dbl[])
      n330 = VISA Clear(VISA resource name=w860) -> (VISA resource name out=w859:refnum<visa-resource-name>, error out=w858:errorcluster)  [unwired: 1 in]
      n331 = property on="Untersetzung-Graph" class="SVDiagr (strikt)"("History Data"=w863) -> ()  [unwired: 2 in, 2 out]
      n332 = VISA Close(VISA resource name=w859, error in (no error)=w858) -> (error out=w857:errorcluster)
      n333 = case shown="Kein Fehler" w857 {
        tunnel: [T4."Enabled" ("Deaktiviert") T4."Disabled and Grayed Out" ("Deaktiviert")] -> w856
        frame No Error {
        }
        frame Error {
        }
      }
      n334 = property on="Start" class="Bool. (strikt)"("DisabledEnum"=w856) -> ()  [unwired: 2 in, 2 out]
    }
  }
  n335 = while {
    stop <- w868 stop-if-true
    n336 = event shown="[3] \"Ende\": Wertänderung" {
      selector: _ -> [_ _ _ _ _ _ _ _]
      dyn-events: _ -> [_ _ _ _ _ _ _ _]
      timeout: _ -> [_ _ _ _ _ _ _ _]
      tunnel: [_ _ _ TRUE _ _ _ _] -> w868
      event "Konfiguration:": Value Change {
        n337 = event-data() -> ("OldVal"=w869:bool)  [unwired: 1 in, 5 out]
        n338 = flat-sequence {
          tunnel: [w873] -> w870
          tunnel: w869 -> [w873]
          tunnel: w870 -> [w899]
          frame #0 {
            n339 = call-poly <vilib>:"Read From XML File.vi"() -> ("error out"=w871:errorcluster, "XML Elements"=w874:string)  [unwired: 9 in, 1 out]
            n340 = property on="Datenspeicher" class="Cluster (strikt)"() -> ("Value"=w872:T3)  [unwired: 2 in, 2 out]
            n341 = case shown="Kein Fehler" w871 {
              selector: w871 -> [_ w898]
              tunnel: w874 -> [w878 _]
              tunnel: w872 -> [w877 _]
              frame No Error {
                n342 = Unflatten From XML(xml string=w878, type=w877) -> (value=w876:T3, error out=w875:errorcluster)  [unwired: 1 in]
                n343 = case shown="Kein Fehler" w875 {
                  tunnel: w876 -> [w896 _]
                  frame No Error {
                    n344 = Unbundle(w896) -> ("Fahrzeugdaten"=w895:string, "Rolle [Inkr/U]"=w894:u16, "Rollenumfang [m]"=w893:dbl, "Rollenträgheit [kgm²]"=w892:dbl, "Zündung [Imp/U]"=w891:dbl, "Getriebe [1:]"=w890:dbl, "Reifenumfang [m]"=w889:dbl, "Gl. Mittelwert"=w888:u8, "Differenzenquotient"=w887:u8, "Lufttemperatur [°C]"=w886:dbl, "Luftfeuchtigkeit [%]"=w885:dbl, "Luftdruck [mbar]"=w884:dbl, "Übersetzung ermitteln aus"=w881:u8, "[s]"=w883:dbl, "n vom Gas [1/min]"=w882:dbl, "Boolesch"=w880:bool, "nKuWe/nRolle"=w879:dbl)  [unwired: 14 out]
                    n345 = property on="Dauer [s]" class="DigWert (strikt)"("Value"=w883) -> ()  [unwired: 2 in, 2 out]
                    n346 = property on="Fahrzeugdaten" class="Str"("Value"=w895) -> ()  [unwired: 2 in, 2 out]
                    n347 = property on="Rollengeber [Inkr/U]" class="DigWert (strikt)"("Value"=w894) -> ()  [unwired: 2 in, 2 out]
                    n348 = property on="Rollenumfang [m]" class="DigWert (strikt)"("Value"=w893) -> ()  [unwired: 2 in, 2 out]
                    n349 = property on="Rollenträgheit [kgm²]" class="DigWert (strikt)"("Value"=w892) -> ()  [unwired: 2 in, 2 out]
                    n350 = property on="Zündung [Imp/U]" class="DigWert (strikt)"("Value"=w891) -> ()  [unwired: 2 in, 2 out]
                    n351 = property on="Getriebe [1:]" class="DigWert (strikt)"("Value"=w890) -> ()  [unwired: 2 in, 2 out]
                    n352 = property on="Reifenumfang [m]" class="DigWert (strikt)"("Value"=w889) -> ()  [unwired: 2 in, 2 out]
                    n353 = property on="Gleitender Mittelwert" class="DigWert (strikt)"("Value"=w888) -> ()  [unwired: 2 in, 2 out]
                    n354 = property on="Differenzenquotient" class="DigWert (strikt)"("Value"=w887) -> ()  [unwired: 2 in, 2 out]
                    n355 = property on="Lufttemperatur [°C]" class="DigWert (strikt)"("Value"=w886) -> ()  [unwired: 2 in, 2 out]
                    n356 = property on="Luftfeuchtigkeit [%]" class="DigWert (strikt)"("Value"=w885) -> ()  [unwired: 2 in, 2 out]
                    n357 = property on="Luftdruck [mbar]" class="DigWert (strikt)"("Value"=w884) -> ()  [unwired: 2 in, 2 out]
                    n358 = property on="Übersetzung ermitteln aus" class="Enum (strikt)"("Val(Sgnl)"=w881) -> ()  [unwired: 2 in, 2 out]
                    n359 = property on="n vom Gas [1/min]" class="DigWert (strikt)"("Value"=w882) -> ()  [unwired: 2 in, 2 out]
                    n360 = property on="Messung Klimadaten" class="Bool. (strikt)"("Val(Sgnl)"=w880) -> ()  [unwired: 2 in, 2 out]
                    n361 = property on="nKuWe/nRolle" class="DigWert (strikt)"("Value"=w879) -> ()  [unwired: 2 in, 2 out]
                  }
                  frame Error {
                    n362 = One Button Dialog(message="Dateiversion nicht kompatibel" ("Nachricht")) -> ()  [unwired: 1 in, 1 out]
                  }
                }
              }
              frame Error {
                n363 = call <vilib>:"Clear Errors.vi"("error in (no error)"=w898) -> ()  [unwired: 5 in, 2 out]
              }
            }
          }
          frame #1 {
            n364 = property on="Konfiguration:" class="Bool. (strikt)"("Value"=w899) -> ()  [unwired: 2 in, 2 out]
          }
        }
      }
      event "Drucken": Value Change {
        n365 = event-data() -> ("OldVal"=w900:bool)  [unwired: 1 in, 5 out]
        n366 = flat-sequence {
          tunnel: [w905] -> w901
          tunnel: w900 -> [w905]
          tunnel: w901 -> [w906]
          frame #0 {
            n367 = control-ref of="Fahrzeugdaten"() -> (w903:refnum<vi>)
            n368 = control-ref of="XY-Graph"() -> (w904:refnum<vi>)
            n369 = control-ref of="Ergebnis"() -> (w902:refnum<vi>)
            n370 = call "printgraph_V0.01.vi"("reference 2"=w902, "Fahrzeugdaten"=w903, "XYGraph (Eingang)"=w904) -> ()  [unwired: 9 in]
          }
          frame #1 {
            n371 = property on="Drucken" class="Bool. (strikt)"("Value"=w906) -> ()  [unwired: 2 in, 2 out]
          }
        }
      }
      event "Speichern": Value Change {
        n372 = event-data() -> ("OldVal"=w908:bool)  [unwired: 1 in, 5 out]
        n373 = control-ref of="Datenspeicher"() -> (w907:refnum<vi>)
        n374 = local write "Speichern"(w908) -> ()
        n375 = call "savecluster_V0.01.vi"("Datenspeicher 3"=w907) -> ()  [unwired: 2 in]
      }
      event "Ende": Value Change {
        w910 = 0.0 ("element")
        (unwired) 0.0 ("element")
        n376 = event-data() -> ("OldVal"=w940:bool)  [unwired: 1 in, 5 out]
        n377 = local write "Ende"(w940) -> ()
        n378 = local read "Datenspeicher"() -> (w911:T3)
        n379 = Unbundle By Name(w911) -> ("Rolle [Inkr/U]"=w932:u16, "Rollenumfang [m]"=w931:dbl, "Rollenträgheit [kgm²]"=w930:dbl, "Zündung [Imp/U]"=w929:dbl, "Getriebe [1:]"=w928:dbl, "Reifenumfang [m]"=w927:dbl, "Gl. Mittelwert"=w926:u8, "Differenzenquotient"=w925:u8, "Polynom"=w924:u8, "Lufttemperatur [°C]"=w923:dbl, "Luftfeuchtigkeit [%]"=w922:dbl, "Luftdruck [mbar]"=w920:dbl, "Best Polynomial Fit"=w921:dbl[], "Übersetzung ermitteln aus"=w919:u8, "[s]"=w918:dbl, "nmin [1/min]"=w917:dbl, "nmax [1/min]"=w916:dbl, "n vom Gas [1/min]"=w915:dbl, "Boolesch"=w914:bool, "Serielle Schnittstelle"=w909:refnum<visa-resource-name>)  [unwired: 3 out]
        n380 = call <vilib>:"Application Directory.vi"() -> ("Application Directory"=w937:path)
        n381 = Bundle By Name(cluster=w911, "Fahrzeugdaten"="", "date/time string"="", "Rolle [Inkr/U]"=w932, "Rollenumfang [m]"=w931, "Rollenträgheit [kgm²]"=w930, "Zündung [Imp/U]"=w929, "Getriebe [1:]"=w928, "Reifenumfang [m]"=w927, "element"=0.0, "Gl. Mittelwert"=w926, "Differenzenquotient"=w925, "Polynom"=w924, "element"=w910, "element"=w910, "Lufttemperatur [°C]"=w923, "Luftfeuchtigkeit [%]"=w922, "Luftdruck [mbar]"=w920, "Best Polynomial Fit"=w921, "Übersetzung ermitteln aus"=w919, "[s]"=w918, "nmin [1/min]"=w917, "nmax [1/min]"=w916, "n vom Gas [1/min]"=w915, "Boolesch"=w914, "Serielle Schnittstelle"=w909) -> (w912:T3)
        n382 = Build Path(base path=w937, name or relative path="Konfig.xml") -> (appended path=w935:path)
        n383 = Flatten To XML(anything=w912) -> (xml string=w939:string)
        n384 = call-poly <vilib>:"Write to XML File.vi"("XML Input"=w939, "XML File Path"=w935) -> ("error out"=w938:errorcluster)  [unwired: 7 in, 2 out]
        n385 = case shown="Kein Fehler" w938 {
          frame No Error {
          }
          frame Error {
          }
        }
      }
      event "Serielle Schnittstelle": Value Change {
        n386 = event-data() -> ()  [unwired: 1 in, 6 out]
        n387 = property on="Start" class="Bool. (strikt)"("DisabledEnum"=T4."Enabled" ("Deaktiviert")) -> ()  [unwired: 2 in, 2 out]
      }
      event "Messung Klimadaten": Value Change {
        n388 = event-data() -> ("NewVal"=w943:bool)  [unwired: 1 in, 5 out]
        n389 = case shown="True" w943 {
          frame True {
            w944 = T4."Disabled and Grayed Out" ("Deaktiviert")
            n390 = property on="Lufttemperatur [°C]" class="DigWert (strikt)"("DisabledEnum"=w944) -> ()  [unwired: 2 in, 2 out]
            n391 = property on="Luftdruck [mbar]" class="DigWert (strikt)"("DisabledEnum"=w944) -> ()  [unwired: 2 in, 2 out]
            n392 = property on="Luftfeuchtigkeit [%]" class="DigWert (strikt)"("DisabledEnum"=w944) -> ()  [unwired: 2 in, 2 out]
          }
          frame False {
            w945 = T4."Enabled" ("Deaktiviert")
            n393 = property on="Lufttemperatur [°C]" class="DigWert (strikt)"("DisabledEnum"=w945) -> ()  [unwired: 2 in, 2 out]
            n394 = property on="Luftdruck [mbar]" class="DigWert (strikt)"("DisabledEnum"=w945) -> ()  [unwired: 2 in, 2 out]
            n395 = property on="Luftfeuchtigkeit [%]" class="DigWert (strikt)"("DisabledEnum"=w945) -> ()  [unwired: 2 in, 2 out]
          }
        }
      }
      event "Recalc": Value Change {
        n396 = event-data() -> ("OldVal"=w948:bool)  [unwired: 1 in, 5 out]
        n397 = property on="Recalc" class="Bool. (strikt)"("Value"=w948) -> ()  [unwired: 2 in, 2 out]
        n398 = property on="Datenspeicher" class="Cluster (strikt)"() -> ("Value"=w946:T3)  [unwired: 2 in, 2 out]
        n399 = call "ReCalc_V2.00.vi"("Berechnen"=TRUE, "Datenspeicher"=w946) -> ()  [unwired: 3 in]
      }
      event "Übersetzung ermitteln aus": Value Change {
        n400 = event-data() -> ("NewVal"=w950:T2)  [unwired: 1 in, 5 out]
        n401 = case shown="\"nKuWe / nRolle\"" w950 {
          tunnel: [T4."Disabled and Grayed Out" ("Deaktiviert") T4."Disabled and Grayed Out" ("Deaktiviert") T4."Enabled" ("Deaktiviert")] -> w952
          frame "nKuWe / nRolle" {
          }
          frame "Zündsignal", Default {
          }
          frame "Getriebe & Reifen" {
          }
        }
        n402 = case shown="\"Zündsignal\", Standard" w950 {
          tunnel: [T4."Enabled" ("Deaktiviert") T4."Disabled and Grayed Out" ("Deaktiviert") T4."Disabled and Grayed Out" ("Deaktiviert")] -> w951
          frame "nKuWe / nRolle" {
          }
          frame "Zündsignal", Default {
          }
          frame "Getriebe & Reifen" {
          }
        }
        n403 = case shown="\"Zündsignal\", Standard" w950 {
          tunnel: [T4."Disabled and Grayed Out" ("Deaktiviert") T4."Enabled" ("Deaktiviert") T4."Disabled and Grayed Out" ("Deaktiviert")] -> w949
          frame "nKuWe / nRolle" {
          }
          frame "Zündsignal", Default {
          }
          frame "Getriebe & Reifen" {
          }
        }
        n404 = property on="Getriebe [1:]" class="DigWert (strikt)"("DisabledEnum"=w952) -> ()  [unwired: 2 in, 2 out]
        n405 = property on="Reifenumfang [m]" class="DigWert (strikt)"("DisabledEnum"=w952) -> ()  [unwired: 2 in, 2 out]
        n406 = property on="nKuWe/nRolle" class="DigWert (strikt)"("DisabledEnum"=w951) -> ()  [unwired: 2 in, 2 out]
        n407 = property on="Dauer [s]" class="DigWert (strikt)"("DisabledEnum"=w949) -> ()  [unwired: 2 in, 2 out]
        n408 = property on="Zündung [Imp/U]" class="DigWert (strikt)"("DisabledEnum"=w949) -> ()  [unwired: 2 in, 2 out]
      }
    }
    n409 = Quit LabVIEW(quit? (T)=w868) -> ()
  }
